vi "Player Info.vi"(11 "Test in":refnum<class "Swarm.lvclass">) -> (0 "Defeat Speech":string, 1 "Victory Speech":string, 2 "Name":string, 3 "Test out":refnum<class "Swarm.lvclass">)   [LabVIEW 2017, in "Swarm.lvclass"]
uses:
  Swarm.lvclass
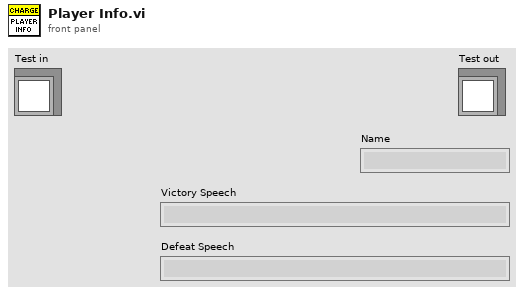
[diagram p1: front panel]
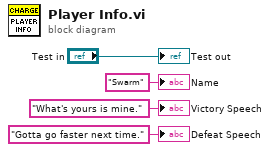
[diagram p0: block diagram]
diagram:
  "Test out" <- "Test in"
  "Name" <- "Swarm" ("Name")
  "Victory Speech" <- "What's yours is mine." ("Victory Speech")
  "Defeat Speech" <- "Gotta go faster next time." ("Defeat Speech")
